vi "欧姆龙PLC通讯Fans UDP-写PLC寄存器.vi"(8 "写入数据编码":string, 9 "端口Port":u16, 10 "IP地址":u32, 11 "UDP网络连接输入":refnum<k16>) -> (1 "布尔":bool, 2 "data out":string, 3 "UDP网络连接输出":refnum<k16>)   [LabVIEW 2014]
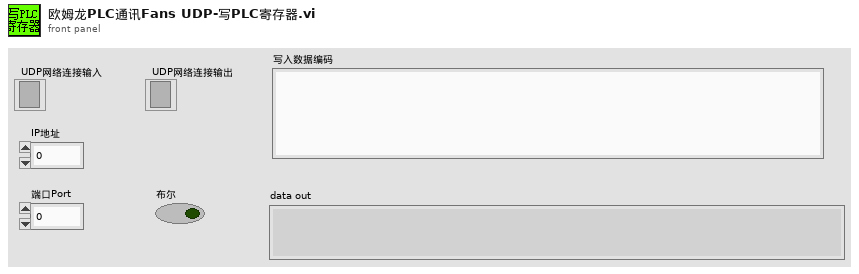
[diagram p1: front panel]
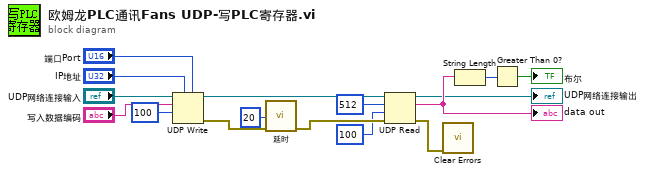
[diagram p0: block diagram]
diagram:
  n1 = UDP Write(address="IP地址", port or service name="端口Port", connection ID="UDP网络连接输入", data in="写入数据编码", 9:100 ("超时毫秒(25000)")) -> (error out=w10:errorcluster, 3:w12:refnum<k16>)  [unwired: 1 in]
  n2 = call "延时.vi"("错误in"=w10, "等待时间（毫秒）"=u32 20) -> ("错误in"=w11:errorcluster)  [unwired: 9 in]
  n3 = UDP Read(connection ID=w12, max size (548)=512 ("读取的字节"), timeout ms (25000)=100 ("超时毫秒(25000)"), 8:w11) -> (data out=w16:string, error out=w1:errorcluster, 3:→"UDP网络连接输出":refnum<k16>)  [unwired: 2 out]
  "data out" <- w16
  n4 = call <vilib>:"Clear Errors.vi"("error in (no error)"=w1) -> ()  [unwired: 5 in, 2 out]
  n5 = String Length(string=w16) -> (length=w5:i32)
  n6 = Greater Than 0?(x=w5) -> (x > 0?=→"布尔":bool)
